vi "Create64PadArray.vi"(8 "Pads 49-64":T4, 9 "Pads 33-48":T2, 10 "Pads 17-32":T6, 11 "Pads 1-16":T8) -> (3 "Pads 1-64":T1(array[cluster]))   [LabVIEW 2012, in "Virtual-PGA.lvlib"]
doc: "This VI converts four groups of 16 pads into one boolean array from 1 to 64 pads."
uses:
  Virtual-PGA.lvlib
  Public/Controls/64PinPGAPads1-16.ctl
  Public/Controls/64PinPGAPad1-16.ctl
  Public/Controls/64PinPGAPads17-32.ctl
  Public/Controls/64PinPGAPad17-32.ctl
  Public/Controls/64PinPGAPads49-64.ctl
  Public/Controls/64PinPGAPad49-64.ctl
  Public/Controls/64PinPGAPads33-48.ctl
  Public/Controls/64PinPGAPad33-48.ctl
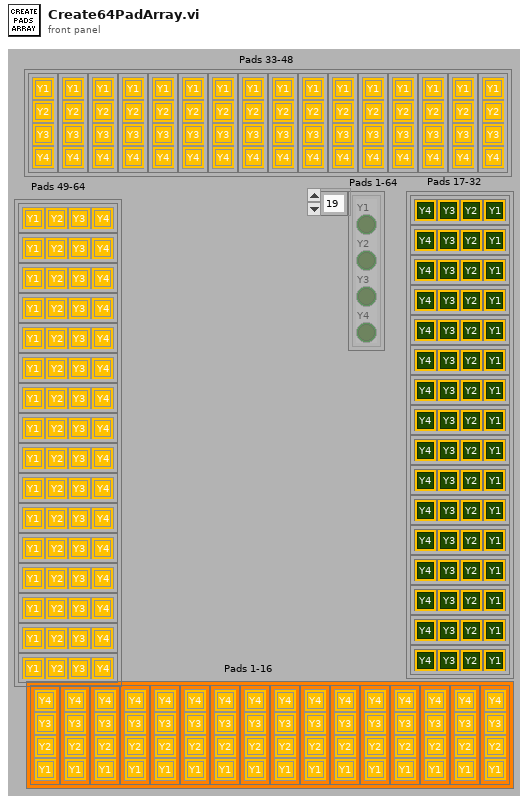
[diagram p1: front panel]
types:
  T1 = cluster{"Y1":bool, "Y2":bool, "Y3":bool, "Y4":bool}[]
  T2 = typedef "Virtual-PGA.lvlib/64PinPGAPads33-48.ctl" = T3[]
  T3 = typedef "Virtual-PGA.lvlib/64PinPGAPad33-48.ctl" = cluster{"Y1":bool, "Y2":bool, "Y3":bool, "Y4":bool}
  T4 = typedef "Virtual-PGA.lvlib/64PinPGAPads49-64.ctl" = T5[]
  T5 = typedef "Virtual-PGA.lvlib/64PinPGAPad49-64.ctl" = cluster{"Y1":bool, "Y2":bool, "Y3":bool, "Y4":bool}
  T6 = typedef "Virtual-PGA.lvlib/64PinPGAPads17-32.ctl" = T7[]
  T7 = typedef "Virtual-PGA.lvlib/64PinPGAPad17-32.ctl" = cluster{"Y1":bool, "Y2":bool, "Y3":bool, "Y4":bool}
  T8 = typedef "Virtual-PGA.lvlib/64PinPGAPads1-16.ctl" = T9[]
  T9 = typedef "Virtual-PGA.lvlib/64PinPGAPad1-16.ctl" = cluster{"Y1":bool, "Y2":bool, "Y3":bool, "Y4":bool}
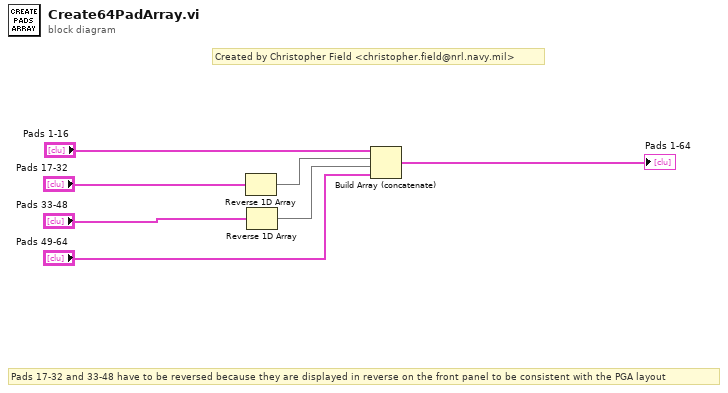
[diagram p0: block diagram]
diagram:
  # "Created by Christopher Field <christopher.field@nrl.navy.mil>"
  # "Pads 17-32 and 33-48 have to be reversed because they are displayed in reverse on the front panel to be consistent with the PGA layout"
  n1 = Reverse 1D Array(array="Pads 17-32") -> (reversed array=w2:T6)
  n2 = Reverse 1D Array(array="Pads 33-48") -> (reversed array=w1:T2)
  n3 = Build Array (concatenate)("Pads 1-16", w2, w1, "Pads 49-64") -> (→"Pads 1-64":T4)
